vi "oa_TV Calculate Continuous Angular Speed (NChan).vi"(6 "pulse/revolution (1)":i32[](array[numeric]), 7 "reset? (False)":bool, 8 "error in (no error)":errorcluster, 9 "filter coefficients":dbl[](array[numeric])=[1.0, 1.0, 1.0] format="%.2f", 10 "deltaX":dbl[](array[numeric]), 11 "Y[n]":cluster{dbl[]}[](array[cluster]) {"?" format="%.2f"}) -> (0 "error out":errorcluster, 2 "dY[n]/dX[n]":cluster{dbl[]}[](array[cluster]), 3 "pulse out":cluster{dbl[]}[](array[cluster]))   [LabVIEW 2017, in "SoundVib_Torsional.lvlib"]
uses:
  <vilib>/addons/Sound and Vibration/Order Analysis/Torsional Vibration/SoundVib_Torsional.lvlib
  <vilib>/Analysis/3filter.llb/FIR Filter with I.C. (DBL).vi
  <vilib>/Analysis/NI_AALBase.lvlib
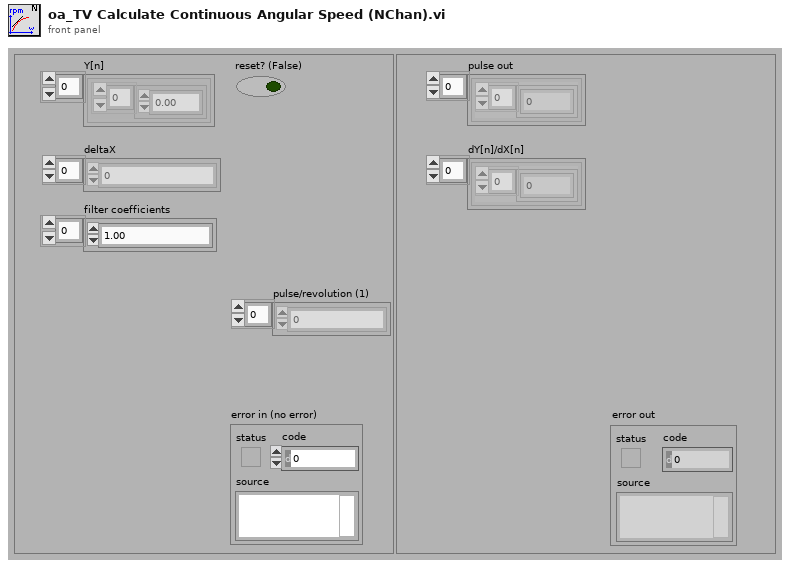
[diagram p1: front panel]
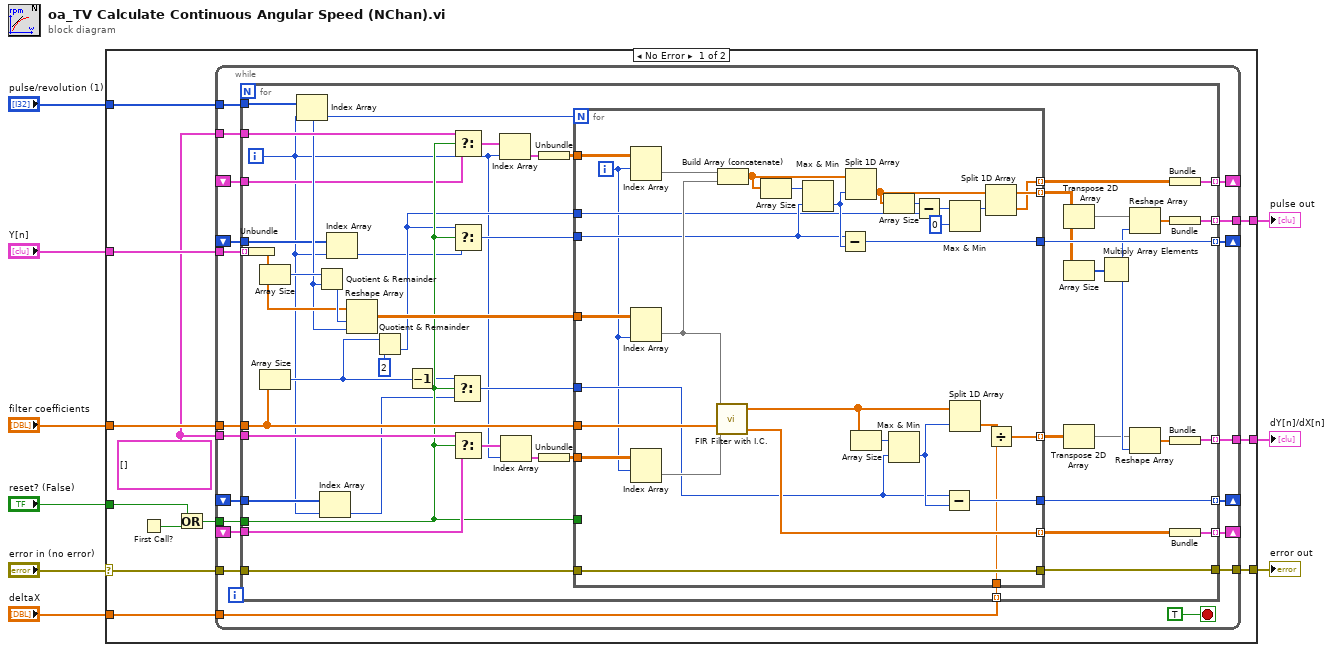
[diagram p0: block diagram]
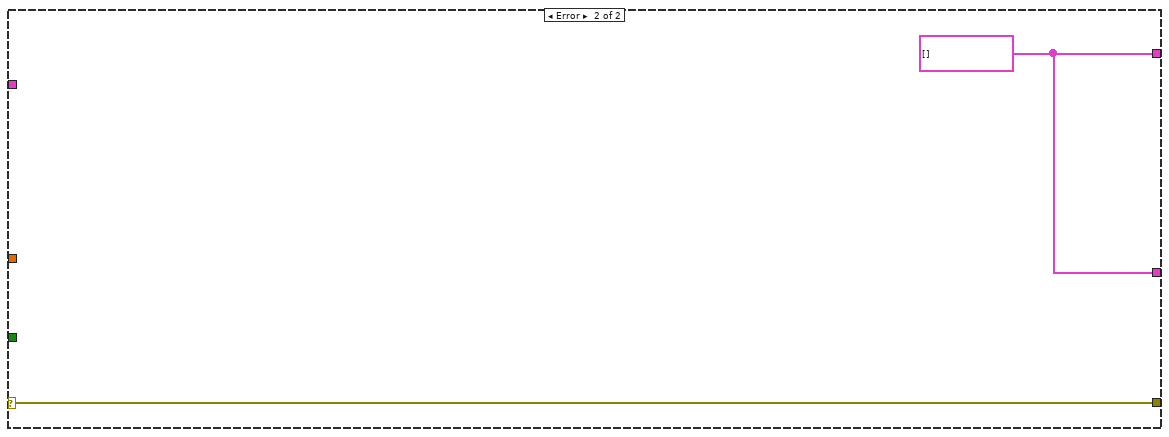
[diagram p2: hidden frame]
diagram:
  n1 = case shown="No Error" "error in (no error)" {
    selector: "error in (no error)" -> [w21 w123]
    tunnel: [w19 w123] -> w6
    tunnel: "Y[n]" -> [w16 _]
    tunnel: "filter coefficients" -> [w20 _]
    tunnel: "reset? (False)" -> [w15 _]
    tunnel: "pulse/revolution (1)" -> [w18 _]
    tunnel: [w17 w122] -> w3
    tunnel: [w11 w122] -> w2
    tunnel: "deltaX" -> [w10 _]
    frame No Error {
      w12 = cluster{dbl[][]}[] []
      n2 = First Call?() -> (First Call?: T/F=w13:bool)
      n3 = Or(x=w15, y=w13) -> (x .or. y?=w14:bool)
      n4 = while {
        tunnel: w21 -> [w41]
        tunnel: w20 -> [w30]
        shift-right: [w23] -> _
        shift-left: _ -> [w35]
        shift-right: [w24] -> _
        shift-left: _ -> [w39]
        shift-right: [w28] -> _
        shift-left: _ -> [w25]
        tunnel: w14 -> [w37]
        tunnel: w12 -> [w38]
        shift-right: [w27] -> _
        shift-left: _ -> [w26]
        tunnel: w12 -> [w36]
        tunnel: w16 -> [w29]
        tunnel: [w34] -> w19
        tunnel: w18 -> [w33]
        tunnel: [w32] -> w17
        tunnel: [w31] -> w11
        tunnel: w10 -> [w22]
        stop <- TRUE stop-if-true
        n5 = for {
          tunnel: w41 -> [w90]
          tunnel: w30 -> [w65]
          tunnel: [w89] -> w28 mode=indexing
          tunnel: [w88] -> w27 mode=indexing
          tunnel: w25 -> [w46]
          tunnel: [w60] -> w24 mode=indexing
          tunnel: w39 -> [w57]
          tunnel: w38 -> [w87]
          tunnel: w37 -> [w64]
          tunnel: w36 -> [w86]
          tunnel: w35 -> [w85]
          tunnel: w29 -> [w70] mode=indexing
          tunnel: [w58] -> w23 mode=indexing
          tunnel: [w84] -> w34
          tunnel: [w76] -> w32 mode=indexing
          tunnel: w33 -> [w68]
          tunnel: [w74] -> w31 mode=indexing
          tunnel: w26 -> [w44]
          tunnel: w22 -> [w47] mode=indexing
          i -> [w43]
          n6 = Unbundle(w70) -> (w71:dbl[])
          n7 = Array Size(array=w71) -> (size(s)=w73:i32)
          n8 = Array Size(array=w65) -> (size(s)=w48:i32)
          n9 = Index Array(array=w68, index=w43) -> (element=w67:i32)
          n10 = Quotient & Remainder(x=w73, y=w67) -> (floor(x/y)=w72:i32)  [unwired: 1 out]
          n11 = Index Array(array=w44, index=w43) -> (element=w42:i32)
          n12 = Index Array(array=w46, index=w43) -> (element=w45:i32)
          n13 = Reshape Array(w71, w72, w67) -> (w69:dbl[][])
          n14 = Quotient & Remainder(x=w48, y=2) -> (floor(x/y)=w49:i32)  [unwired: 1 out]
          n15 = Decrement(x=w48) -> (x-1=w50:i32)
          n16 = Select(t=w50, s=w64, f=w42) -> (s? t:f=w62:i32)
          n17 = Select(t=w87, s=w64, f=w57) -> (s? t:f=w56:cluster{dbl[][]}[])
          n18 = Select(t=w49, s=w64, f=w45) -> (s? t:f=w63:i32)
          n19 = Select(t=w86, s=w64, f=w85) -> (s? t:f=w52:cluster{"Final X Conditions":dbl[][]}[])
          n20 = Index Array(array=w56, index=w43) -> (element=w55:cluster{dbl[][]})
          n21 = Index Array(array=w52, index=w43) -> (element=w53:cluster{"Final X Conditions":dbl[][]})
          n22 = Unbundle(w55) -> (w54:dbl[][])
          n23 = Unbundle(w53) -> ("Final X Conditions"=w51:dbl[][])
          n24 = for {
            N: w67 -> [_]
            tunnel: [w121] -> w78 mode=indexing
            tunnel: w90 -> [w99]
            tunnel: w65 -> [w104]
            tunnel: [w118] -> w89
            tunnel: [w113] -> w79 mode=indexing
            tunnel: [w110] -> w88
            tunnel: w64 -> [_]
            tunnel: [w107] -> w61 mode=indexing
            tunnel: w69 -> [w106]
            tunnel: [w101] -> w59 mode=indexing
            tunnel: [w99] -> w84
            tunnel: w63 -> [w98]
            tunnel: w49 -> [w97]
            tunnel: w62 -> [w96]
            tunnel: w54 -> [w94]
            tunnel: w51 -> [w93]
            tunnel: w47 -> [w91]
            i -> [w92]
            n25 = Index Array(array=w94, index (row)=w92) -> (element=w95:dbl[])  [unwired: 1 in]
            n26 = Index Array(array=w106, index (col)=w92) -> (element=w105:dbl[])  [unwired: 1 in]
            n27 = Index Array(array=w93, index (row)=w92) -> (element=w100:dbl[])  [unwired: 1 in]
            n28 = call-poly <vilib>:"FIR Filter with I.C..vi"("Initial X Conditions"=w100, "FIR Coefficients"=w104, "X"=w105) -> ("Final X Conditions"=w101:dbl[], "Filtered X"=w102:dbl[])  [unwired: 5 in, 1 out]
            n29 = Build Array (concatenate)(w95, w105) -> (w108:dbl[])
            n30 = Array Size(array=w108) -> (size(s)=w120:i32)
            n31 = Max & Min(x=w120, y=w98) -> (min(x,y)=w119:i32)  [unwired: 1 out]
            n32 = Subtract(x=w98, y=w119) -> (x-y=w118:i32)
            n33 = Split 1D Array(array=w108, index=w119) -> (second subarray=w117:dbl[])  [unwired: 1 out]
            n34 = Array Size(array=w102) -> (size(s)=w112:i32)
            n35 = Array Size(array=w117) -> (size(s)=w116:i32)
            n36 = Max & Min(x=w112, y=w96) -> (min(x,y)=w111:i32)  [unwired: 1 out]
            n37 = Subtract(x=w116, y=w97) -> (x-y=w115:i32)
            n38 = Subtract(x=w96, y=w111) -> (x-y=w110:i32)
            n39 = Max & Min(x=w115, y=0) -> (max(x,y)=w109:i32)  [unwired: 1 out]
            n40 = Split 1D Array(array=w102, index=w111) -> (second subarray=w103:dbl[])  [unwired: 1 out]
            n41 = Split 1D Array(array=w117, index=w109) -> (first subarray=w113:dbl[], second subarray=w107:dbl[])
            n42 = Divide(x=w103, y=w91) -> (x/y=w121:dbl[])
          }
          n43 = Transpose 2D Array(2D array=w79) -> (transposed array=w80:dbl[][])
          n44 = Array Size(array=w79) -> (size(s)=w81:i32[])
          n45 = Transpose 2D Array(2D array=w78) -> (transposed array=w82:dbl[][])
          n46 = Multiply Array Elements(1:w81) -> (0:w83:i32)
          n47 = Reshape Array(w80, w83) -> (w77:dbl[])
          n48 = Reshape Array(w82, w83) -> (w75:dbl[])
          n49 = Bundle(w61) -> (w60:cluster{dbl[][]})  [unwired: 1 in]
          n50 = Bundle(w77) -> (w76:cluster{dbl[]})  [unwired: 1 in]
          n51 = Bundle(w75) -> (w74:cluster{dbl[]})  [unwired: 1 in]
          n52 = Bundle("Final X Conditions"=w59) -> (w58:cluster{"Final X Conditions":dbl[][]})  [unwired: 1 in]
        }
      }
    }
    frame Error {
      w122 = cluster{dbl[]}[] []
    }
  }
  "error out" <- w6
  "pulse out" <- w3
  "dY[n]/dX[n]" <- w2
